vi "CIF proto Pre-Uninstall Custom Action.vi"(10 "Variant":variant) -> (0 "error out":errorcluster)   [LabVIEW 2021]
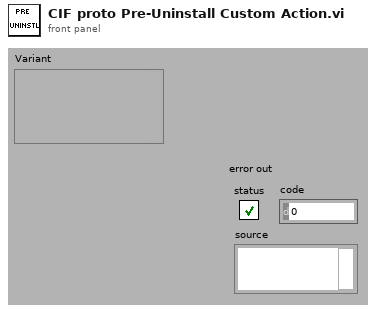
[diagram p1: front panel]
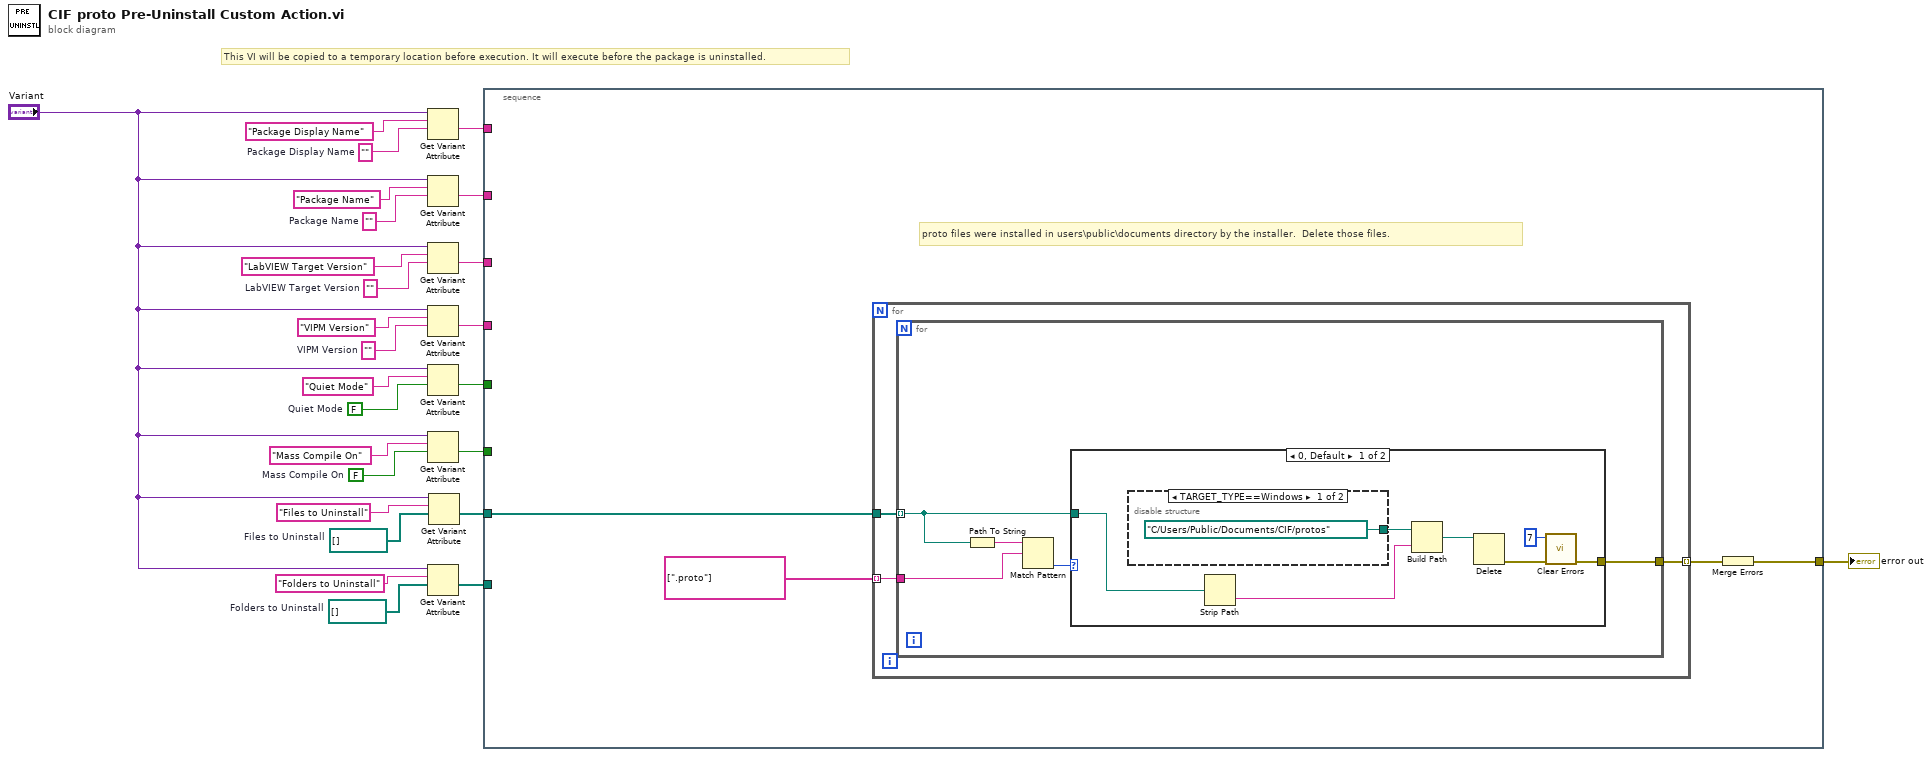
[diagram p0: block diagram]
diagram:
  w4 = path[] []  # Folders to Uninstall
  w8 = path[] []  # Files to Uninstall
  w9 = FALSE  # Mass Compile On
  w10 = ""  # Package Display Name
  w17 = FALSE  # Quiet Mode
  w20 = ""  # VIPM Version
  w22 = ""  # LabVIEW Target Version
  w24 = ""  # Package Name
  # "This VI will be copied to a temporary location before execution. It will execute before the package is uninstalled."
  n1 = Get Variant Attribute(Variant="Variant", name="Package Display Name", default value (empty Variant)=w10) -> (value=w16:string)  [unwired: 1 in, 3 out]
  n2 = Get Variant Attribute(Variant="Variant", name="Package Name", default value (empty Variant)=w24) -> (value=w15:string)  [unwired: 1 in, 3 out]
  n3 = Get Variant Attribute(Variant="Variant", name="LabVIEW Target Version", default value (empty Variant)=w22) -> (value=w14:string)  [unwired: 1 in, 3 out]
  n4 = Get Variant Attribute(Variant="Variant", name="VIPM Version", default value (empty Variant)=w20) -> (value=w13:string)  [unwired: 1 in, 3 out]
  n5 = Get Variant Attribute(Variant="Variant", name="Quiet Mode", default value (empty Variant)=w17) -> (value=w12:bool)  [unwired: 1 in, 3 out]
  n6 = Get Variant Attribute(Variant="Variant", name="Mass Compile On", default value (empty Variant)=w9) -> (value=w11:bool)  [unwired: 1 in, 3 out]
  n7 = Get Variant Attribute(Variant="Variant", name="Folders to Uninstall", default value (empty Variant)=w4) -> (value=w3:path[])  [unwired: 1 in, 3 out]
  n8 = Get Variant Attribute(Variant="Variant", name="Files to Uninstall", default value (empty Variant)=w8) -> (value=w6:path[])  [unwired: 1 in, 3 out]
  n9 = stacked-sequence {
    tunnel: w16 -> [_]
    tunnel: w15 -> [_]
    tunnel: w14 -> [_]
    tunnel: w13 -> [_]
    tunnel: w12 -> [_]
    tunnel: w11 -> [_]
    tunnel: w6 -> [w28]
    tunnel: w3 -> [_]
    tunnel: [w27] -> w1
    frame #0 {
      # "proto files were installed in users\\public\\documents directory by the installer.  Delete those files."
      n10 = for {
        tunnel: w28 -> [w33]
        tunnel: string[] [".proto"] -> [w32] mode=indexing
        tunnel: [w31] -> w29 mode=indexing
        n11 = for {
          tunnel: w33 -> [w36] mode=indexing
          tunnel: w32 -> [w35]
          tunnel: [w34] -> w31
          n12 = Path To String(path=w36) -> (string=w38:string)
          n13 = Match Pattern(string=w38, regular expression=w35) -> (offset past match=w37:i32)  [unwired: 1 in, 3 out]
          n14 = case shown="0, Default" w37 {
            tunnel: w36 -> [w44 _]
            tunnel: [w40 _] -> w34
            frame 0, Default {
              n15 = disable-structure shown="TARGET_TYPE==Windows" {
                disable-tunnel: [path "C:/Users/Public/Documents/CIF/protos" ("configuration file path") _] -> w42
                frame condition #0 (active) {
                }
                frame condition #1 {
                }
              }
              n16 = Strip Path(path=w44) -> (name=w45:string)  [unwired: 1 out]
              n17 = Build Path(base path=w42, name or relative path=w45) -> (appended path=w43:path)
              n18 = Delete(path (use dialog)=w43) -> (error out=w41:errorcluster)  [unwired: 4 in, 2 out]
              n19 = call <vilib>:"Clear Errors.vi"("error in (no error)"=w41, "specific error code to clear (0: all)"=7) -> ("error out"=w40:errorcluster)  [unwired: 4 in, 1 out]
            }
            frame -1 {
            }
          }
        }
      }
      n20 = Merge Errors(w29) -> (w27:errorcluster)
    }
  }
  "error out" <- w1
